vi "Constant Loader.vi"() -> ()   [LabVIEW 2014]
uses:
  <vilib>/regexp/Match Regular Expression.xnode
  Type Defs/Definition.ctl
  Sensors/VL6180/VL6180X DEFS.ctl
panel:
  in  "VL6180X Constants":T1 items=["IDENTIFICATION_MODEL_ID"=0, "IDENTIFICATION_MODEL_REV_MAJOR"=1, "IDENTIFICATION_MODEL_REV_MINOR"=2, "IDENTIFICATION_MODULE_REV_MAJOR"=3, "IDENTIFICATION_MODULE_REV_MINOR"=4, "IDENTIFICATION_DATE"=6, "IDENTIFICATION_TIME"=8, "SYSTEM_MODE_GPIO0"=16, "SYSTEM_MODE_GPIO1"=17, "SYSTEM_HISTORY_CTRL"=18, "SYSTEM_INTERRUPT_CONFIG_GPIO"=20, "SYSTEM_INTERRUPT_CLEAR"=21, "SYSTEM_FRESH_OUT_OF_RESET"=22, "SYSTEM_GROUPED_PARAMETER_HOLD"=23, "SYSRANGE_START"=24, "SYSRANGE_THRESH_HIGH"=25, "SYSRANGE_THRESH_LOW"=26, "SYSRANGE_INTERMEASUREMENT_PERIOD"=27, "SYSRANGE_MAX_CONVERGENCE_TIME"=28, "SYSRANGE_CROSSTALK_COMPENSATION_RATE"=30, "SYSRANGE_CROSSTALK_VALID_HEIGHT"=33, "SYSRANGE_EARLY_CONVERGENCE_ESTIMATE"=34, "SYSRANGE_PART_TO_PART_RANGE_OFFSET"=36, "SYSRANGE_RANGE_IGNORE_VALID_HEIGHT"=37, "SYSRANGE_RANGE_IGNORE_THRESHOLD"=38, "SYSRANGE_MAX_AMBIENT_LEVEL_MULT"=44, "SYSRANGE_RANGE_CHECK_ENABLES"=45, "SYSRANGE_VHV_RECALIBRATE"=46, "SYSRANGE_VHV_REPEAT_RATE"=49, "SYSALS_START"=56, "SYSALS_THRESH_HIGH"=58, "SYSALS_THRESH_LOW"=60, "SYSALS_INTERMEASUREMENT_PERIOD"=62, "SYSALS_ANALOGUE_GAIN"=63, "SYSALS_INTEGRATION_PERIOD"=64, "RESULT_RANGE_STATUS"=77, "RESULT_ALS_STATUS"=78, "RESULT_INTERRUPT_STATUS_GPIO"=79, "RESULT_ALS_VAL"=80, "RESULT_HISTORY_BUFFER"=82, "RESULT_RANGE_VAL"=98, "RESULT_RANGE_RAW"=100, "RESULT_RANGE_RETURN_RATE"=102, "RESULT_RANGE_REFERENCE_RATE"=104, "RESULT_RANGE_RETURN_SIGNAL_COUNT"=108, "RESULT_RANGE_REFERENCE_SIGNAL_COUNT"=112, "RESULT_RANGE_RETURN_AMB_COUNT"=116, "RESULT_RANGE_REFERENCE_AMB_COUNT"=120, "RESULT_RANGE_RETURN_CONV_TIME"=124, "RESULT_RANGE_REFERENCE_CONV_TIME"=128, "READOUT_AVERAGING_SAMPLE_PERIOD"=266, "FIRMWARE_BOOTUP"=281, "FIRMWARE_RESULT_SCALER"=288, "I2C_SLAVE_DEVICE_ADDRESS"=530, "INTERLEAVED_MODE_ENABLE"=675]
  out "CMD":string
  out "Desc":string
  out "V6180X Definitions":T2[](array[typedef])=[{"Desc"="IDENTIFICATION_MODEL_ID", "Hex Command"=0}, {"Desc"="IDENTIFICATION_MODEL_REV_MAJOR", "Hex Command"=1}, {"Desc"="IDENTIFICATION_MODEL_REV_MINOR", "Hex Command"=2}, {"Desc"="IDENTIFICATION_MODULE_REV_MAJOR", "Hex Command"=3}, {"Desc"="IDENTIFICATION_MODULE_REV_MINOR", "Hex Command"=4}, {"Desc"="IDENTIFICATION_DATE", "Hex Command"=6}, {"Desc"="IDENTIFICATION_TIME", "Hex Command"=8}, {"Desc"="SYSTEM_MODE_GPIO0", "Hex Command"=16}, {"Desc"="SYSTEM_MODE_GPIO1", "Hex Command"=17}, {"Desc"="SYSTEM_HISTORY_CTRL", "Hex Command"=18}, {"Desc"="SYSTEM_INTERRUPT_CONFIG_GPIO", "Hex Command"=20}, {"Desc"="SYSTEM_INTERRUPT_CLEAR", "Hex Command"=21}, {"Desc"="SYSTEM_FRESH_OUT_OF_RESET", "Hex Command"=22}, {"Desc"="SYSTEM_GROUPED_PARAMETER_HOLD", "Hex Command"=23}, {"Desc"="SYSRANGE_START", "Hex Command"=24}, {"Desc"="SYSRANGE_THRESH_HIGH", "Hex Command"=25}, {"Desc"="SYSRANGE_THRESH_LOW", "Hex Command"=26}, {"Desc"="SYSRANGE_INTERMEASUREMENT_PERIOD", "Hex Command"=27}, {"Desc"="SYSRANGE_MAX_CONVERGENCE_TIME", "Hex Command"=28}, {"Desc"="SYSRANGE_CROSSTALK_COMPENSATION_RATE", "Hex Command"=30}, {"Desc"="SYSRANGE_CROSSTALK_VALID_HEIGHT", "Hex Command"=33}, {"Desc"="SYSRANGE_EARLY_CONVERGENCE_ESTIMATE", "Hex Command"=34}, {"Desc"="SYSRANGE_PART_TO_PART_RANGE_OFFSET", "Hex Command"=36}, {"Desc"="SYSRANGE_RANGE_IGNORE_VALID_HEIGHT", "Hex Command"=37}, {"Desc"="SYSRANGE_RANGE_IGNORE_THRESHOLD", "Hex Command"=38}, {"Desc"="SYSRANGE_MAX_AMBIENT_LEVEL_MULT", "Hex Command"=44}, {"Desc"="SYSRANGE_RANGE_CHECK_ENABLES", "Hex Command"=45}, {"Desc"="SYSRANGE_VHV_RECALIBRATE", "Hex Command"=46}, {"Desc"="SYSRANGE_VHV_REPEAT_RATE", "Hex Command"=49}, {"Desc"="SYSALS_START", "Hex Command"=56}, {"Desc"="SYSALS_THRESH_HIGH", "Hex Command"=58}, {"Desc"="SYSALS_THRESH_LOW", "Hex Command"=60}, {"Desc"="SYSALS_INTERMEASUREMENT_PERIOD", "Hex Command"=62}, {"Desc"="SYSALS_ANALOGUE_GAIN", "Hex Command"=63}, {"Desc"="SYSALS_INTEGRATION_PERIOD", "Hex Command"=64}, {"Desc"="RESULT_RANGE_STATUS", "Hex Command"=77}, {"Desc"="RESULT_ALS_STATUS", "Hex Command"=78}, {"Desc"="RESULT_INTERRUPT_STATUS_GPIO", "Hex Command"=79}, {"Desc"="RESULT_ALS_VAL", "Hex Command"=80}, {"Desc"="RESULT_HISTORY_BUFFER", "Hex Command"=82}, {"Desc"="RESULT_RANGE_VAL", "Hex Command"=98}, {"Desc"="RESULT_RANGE_RAW", "Hex Command"=100}, {"Desc"="RESULT_RANGE_RETURN_RATE", "Hex Command"=102}, {"Desc"="RESULT_RANGE_REFERENCE_RATE", "Hex Command"=104}, {"Desc"="RESULT_RANGE_RETURN_SIGNAL_COUNT", "Hex Command"=108}, {"Desc"="RESULT_RANGE_REFERENCE_SIGNAL_COUNT", "Hex Command"=112}, {"Desc"="RESULT_RANGE_RETURN_AMB_COUNT", "Hex Command"=116}, {"Desc"="RESULT_RANGE_REFERENCE_AMB_COUNT", "Hex Command"=120}, {"Desc"="RESULT_RANGE_RETURN_CONV_TIME", "Hex Command"=124}, {"Desc"="RESULT_RANGE_REFERENCE_CONV_TIME", "Hex Command"=128}, {"Desc"="READOUT_AVERAGING_SAMPLE_PERIOD", "Hex Command"=266}, {"Desc"="FIRMWARE_BOOTUP", "Hex Command"=281}, {"Desc"="FIRMWARE_RESULT_SCALER", "Hex Command"=288}, {"Desc"="I2C_SLAVE_DEVICE_ADDRESS", "Hex Command"=530}, {"Desc"="INTERLEAVED_MODE_ENABLE", "Hex Command"=675}] {"Hex Command" format="%04x"}
  in  "From SparkFun Documentation":string="#define VL6180X_IDENTIFICATION_MODEL_ID              0x0000\n#define VL6180X_IDENTIFICATION_MODEL_REV_MAJOR       0x0001\n#define VL6180X_IDENTIFICATION_MODEL_REV_MINOR       0x0002\n#define VL6180X_IDENTIFICATION_MODULE_REV_MAJOR      0x0003\n#define VL6180X_IDENTIFICATION_MODULE_REV_MINOR      0x0004\n#define VL6180X_IDENTIFICATION_DATE                  0x0006 //16bit value\n#define VL6180X_IDENTIFICATION_TIME                  0x0008 //16bit value\n#define VL6180X_SYSTEM_MODE_GPIO0                    0x0010\n#define VL6180X_SYSTEM_MODE_GPIO1                    0x0011\n#define VL6180X_SYSTEM_HISTORY_CTRL                  0x0012\n#define VL6180X_SYSTEM_INTERRUPT_CONFIG_GPIO         0x0014\n#define VL6180X_SYSTEM_INTERRUPT_CLEAR               0x0015\n#define VL6180X_SYSTEM_FRESH_OUT_OF_RESET            0x0016\n#define VL6180X_SYSTEM_GROUPED_PARAMETER_HOLD        0x0017\n#define VL6180X_SYSRANGE_START                       0x0018\n#define VL6180X_SYSRANGE_THRESH_HIGH                 0x0019\n#define VL6180X_SYSRANGE_THRESH_LOW                  0x001A\n#define VL6180X_SYSRANGE_INTERMEASUREMENT_PERIOD     0x001B\n#define VL6180X_SYSRANGE_MAX_CONVERGENCE_TIME        0x001C\n#define VL6180X_SYSRANGE_CROSSTALK_COMPENSATION_RATE 0x001E\n#define VL6180X_SYSRANGE_CROSSTALK_VALID_HEIGHT      0x0021\n#define VL6180X_SYSRANGE_EARLY_CONVERGENCE_ESTIMATE  0x0022\n#define VL6180X_SYSRANGE_PART_TO_PART_RANGE_OFFSET   0x0024\n#define VL6180X_SYSRANGE_RANGE_IGNORE_VALID_HEIGHT   0x0025\n#define VL6180X_SYSRANGE_RANGE_IGNORE_THRESHOLD      0x0026\n#define VL6180X_SYSRANGE_MAX_AMBIENT_LEVEL_MULT      0x002C\n#define VL6180X_SYSRANGE_RANGE_CHECK_ENABLES         0x002D\n#define VL6180X_SYSRANGE_VHV_RECALIBRATE             0x002E\n#define VL6180X_SYSRANGE_VHV_REPEAT_RATE             0x0031\n#define VL6180X_SYSALS_START                         0x0038\n#define VL6180X_SYSALS_THRESH_HIGH                   0x003A\n#define VL6180X_SYSALS_THRESH_LOW                    0x003C\n#define VL6180X_SYSALS_INTERMEASUREMENT_PERIOD       0x003E\n#define VL6180X_SYSALS_ANALOGUE_GAIN                 0x003F\n#define VL6180X_SYSALS_INTEGRATION_PERIOD            0x0040\n#define VL6180X_RESULT_RANGE_STATUS                  0x004D\n#define VL6180X_RESULT_ALS_STATUS                    0x004E\n#define VL6180X_RESULT_INTERRUPT_STATUS_GPIO         0x004F\n#define VL6180X_RESULT_ALS_VAL                       0x0050\n#define VL6180X_RESULT_HISTORY_BUFFER                0x0052 \n#define VL6180X_RESULT_RANGE_VAL                     0x0062\n#define VL6180X_RESULT_RANGE_RAW                     0x0064\n#define VL6180X_RESULT_RANGE_RETURN_RATE             0x0066\n#define VL6180X_RESULT_RANGE_REFERENCE_RATE          0x0068\n#define VL6180X_RESULT_RANGE_RETURN_SIGNAL_COUNT     0x006C\n#define VL6180X_RESULT_RANGE_REFERENCE_SIGNAL_COUNT  0x0070\n#define VL6180X_RESULT_RANGE_RETURN_AMB_COUNT        0x0074\n#define VL6180X_RESULT_RANGE_REFERENCE_AMB_COUNT     0x0078\n#define VL6180X_RESULT_RANGE_RETURN_CONV_TIME        0x007C\n#define VL6180X_RESULT_RANGE_REFERENCE_CONV_TIME     0x0080\n#define VL6180X_READOUT_AVERAGING_SAMPLE_PERIOD      0x010A\n#define VL6180X_FIRMWARE_BOOTUP                      0x0119\n#define VL6180X_FIRMWARE_RESULT_SCALER               0x0120\n#define VL6180X_I2C_SLAVE_DEVICE_ADDRESS             0x0212\n#define VL6180X_INTERLEAVED_MODE_ENABLE              0x02A3"
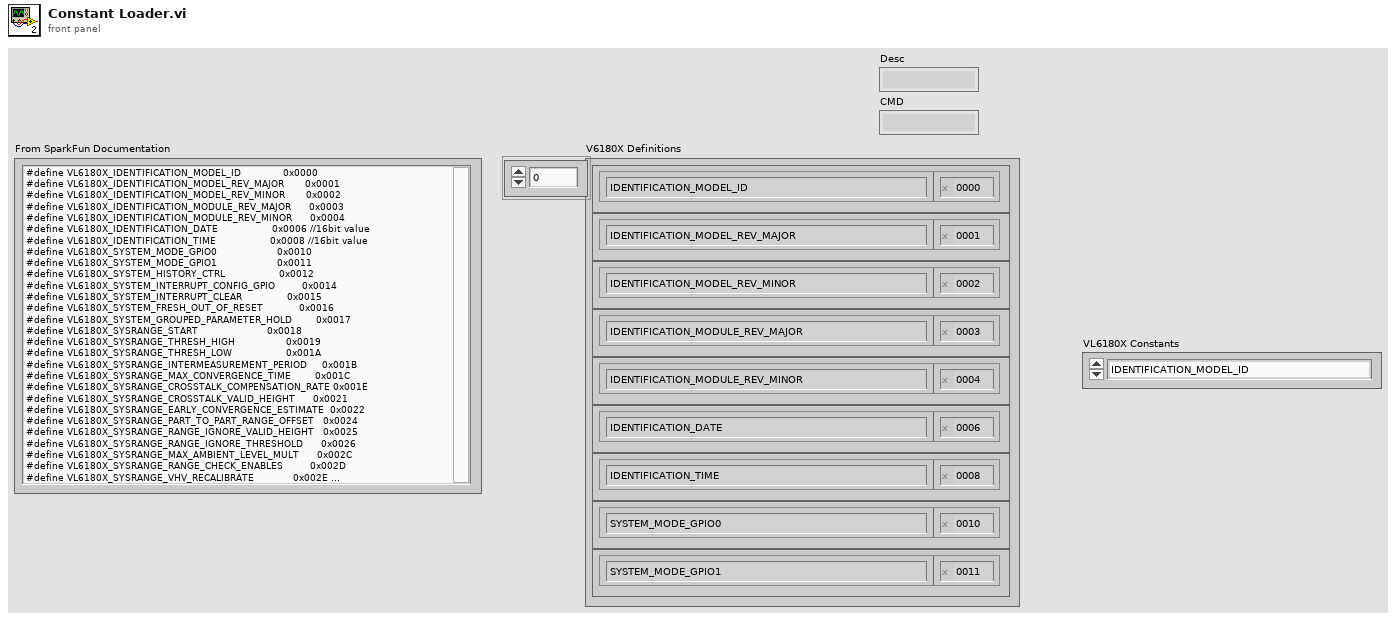
[diagram p1: front panel]
types:
  T1 = typedef "VL6180X DEFS.ctl" = u16
  T2 = typedef "Definition.ctl" = cluster{"Desc":string, "Hex Command":u16}
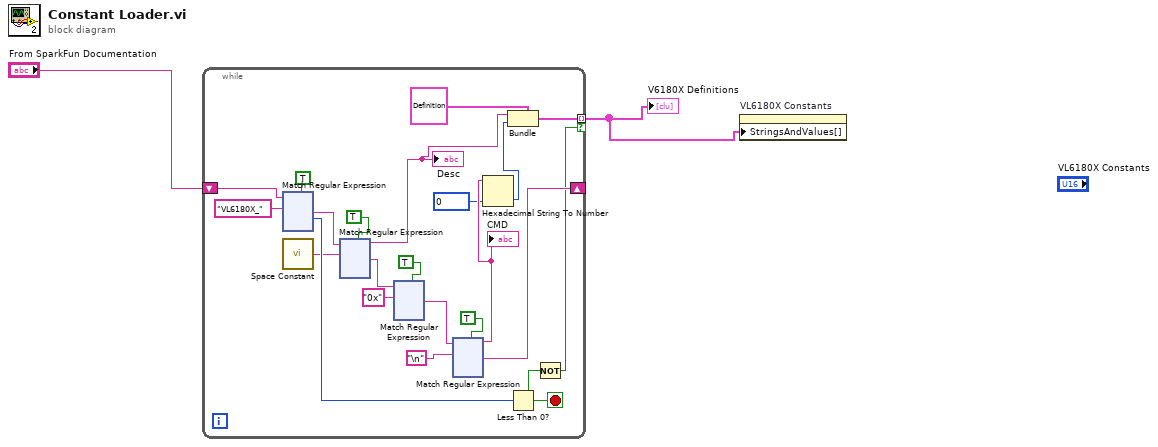
[diagram p0: block diagram]
diagram:
  n1 = while {
    shift-right: [w14] -> _
    shift-left: "From SparkFun Documentation" -> [w23]
    tunnel: [w8] -> w1 mode=indexing if=w3
    stop <- w4 stop-if-true
    n2 = xnode "Match Regular Expression"("input string"=w23, "regular expression"="VL6180X_", "multiline? (F)"=TRUE) -> ("after match"=w20:string, "offset past match"=w24:i32)  [unwired: 3 in, 3 out]
    n3 = call <vilib>:"Space Constant.vi"() -> ("String"=w19:string)
    n4 = xnode "Match Regular Expression"("input string"=w20, "regular expression"=w19, "multiline? (F)"=TRUE) -> ("before match"=w9:string, "after match"=w18:string)  [unwired: 3 in, 3 out]
    "Desc" <- w9
    n5 = xnode "Match Regular Expression"("input string"=w18, "regular expression"="0x", "multiline? (F)"=TRUE) -> ("after match"=w15:string)  [unwired: 3 in, 4 out]
    n6 = xnode "Match Regular Expression"("input string"=w15, "regular expression"="\n", "multiline? (F)"=TRUE) -> ("before match"=w7:string, "after match"=w14:string)  [unwired: 3 in, 3 out]
    "CMD" <- w7
    n7 = Hexadecimal String To Number(string=w7, default (0uL)=u16 0) -> (number=w5:u16)  [unwired: 1 in, 1 out]
    n8 = Bundle(cluster=T2 {"Desc"="VL6180X_RESULT_RANGE_REFERENCE_SIGNAL_COUNT", "Hex Command"=0} ("Constant"), "Desc"=w9, "Hex Command"=w5) -> (w8:T2)
    n9 = Less Than 0?(x=w24) -> (x < 0?=w4:bool)
    n10 = Not(x=w4) -> (.not. x?=w3:bool)
  }
  "V6180X Definitions" <- w1
  n11 = property on="VL6180X Constants" class="Ring (strict)"("StringsAndValues[]"=w1) -> ()  [unwired: 2 in, 2 out]
